vi "Move.vi"(8 "error in (no error)":errorcluster, 11 "IgusMotorDrive in":refnum<class "IgusMotorDrive.lvclass">) -> (0 "error out":errorcluster, 3 "IgusMotorDrive out":refnum<class "IgusMotorDrive.lvclass">)   [LabVIEW 2016, in "IgusMotorDrive.lvclass"]
uses:
  IgusMotorDrive.lvclass
  C:/Users/illogicdev/Desktop/IGUS/IgusPositioningSystem Folder/Modules/Classes/motor-drive/MotorDrive.lvclass
  Libraries/Modbus-Master/MB_PDU/MB_PDU_Cluster.ctl
  typedefs/Controlword--cluster.ctl
  IgusMotorDrive.lvclass/IgusMotorDrive.ctl
  Libraries/Modbus-Master/MB_Master_TCP/MB_Master_TCP.lvclass
  C:/Users/illogicdev/Desktop/IGUS/IgusPositioningSystem Folder/Modules/Libraries/Modbus-Master/MB_Master/MB_Master.lvclass
  motor-drive/MotorDrive.lvclass
  Libraries/Modbus-Master/MB Master.lvlib
panel:
  out "operation mode":u8
  out "Command":T1 {"Data" format="%.0x"}
  out "Response":T1 {"Data" format="%.0x"}
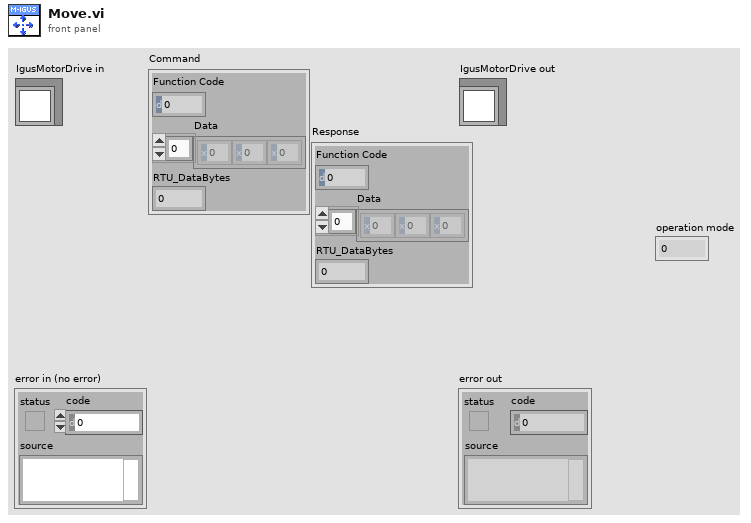
[diagram p1: front panel]
types:
  T1 = typedef "MB Master.lvlib/MB_PDU_Cluster.ctl" = cluster{"Function Code":u8, "Data":u8[], "RTU_DataBytes":i32}
  T2 = typedef "IgusMotorDrive.lvclass/Controlword--cluster.ctl" = cluster{"Switch On":bool, "Enable Voltage":bool, "Quick Stop":bool, "Enable Operation":bool, "4 MS (0: Homing Blocked/1: Homing Start) (0: No Start Signal/1: Start of Movement (0>1))":bool, "5 MS":bool, "6 MS(0:Absolute Positioning/1:Relative Positioning)":bool, "Fault Reset":bool, "Stop":bool, "9 MS":bool, "10 Reserved":bool, "11 Manufacturer Specific":bool, "12 Manufacturer Specific":bool, "13 Manufacturer Specific":bool, "14 Manufacturer Specific":bool, "15 Manufacturer Specific":bool}
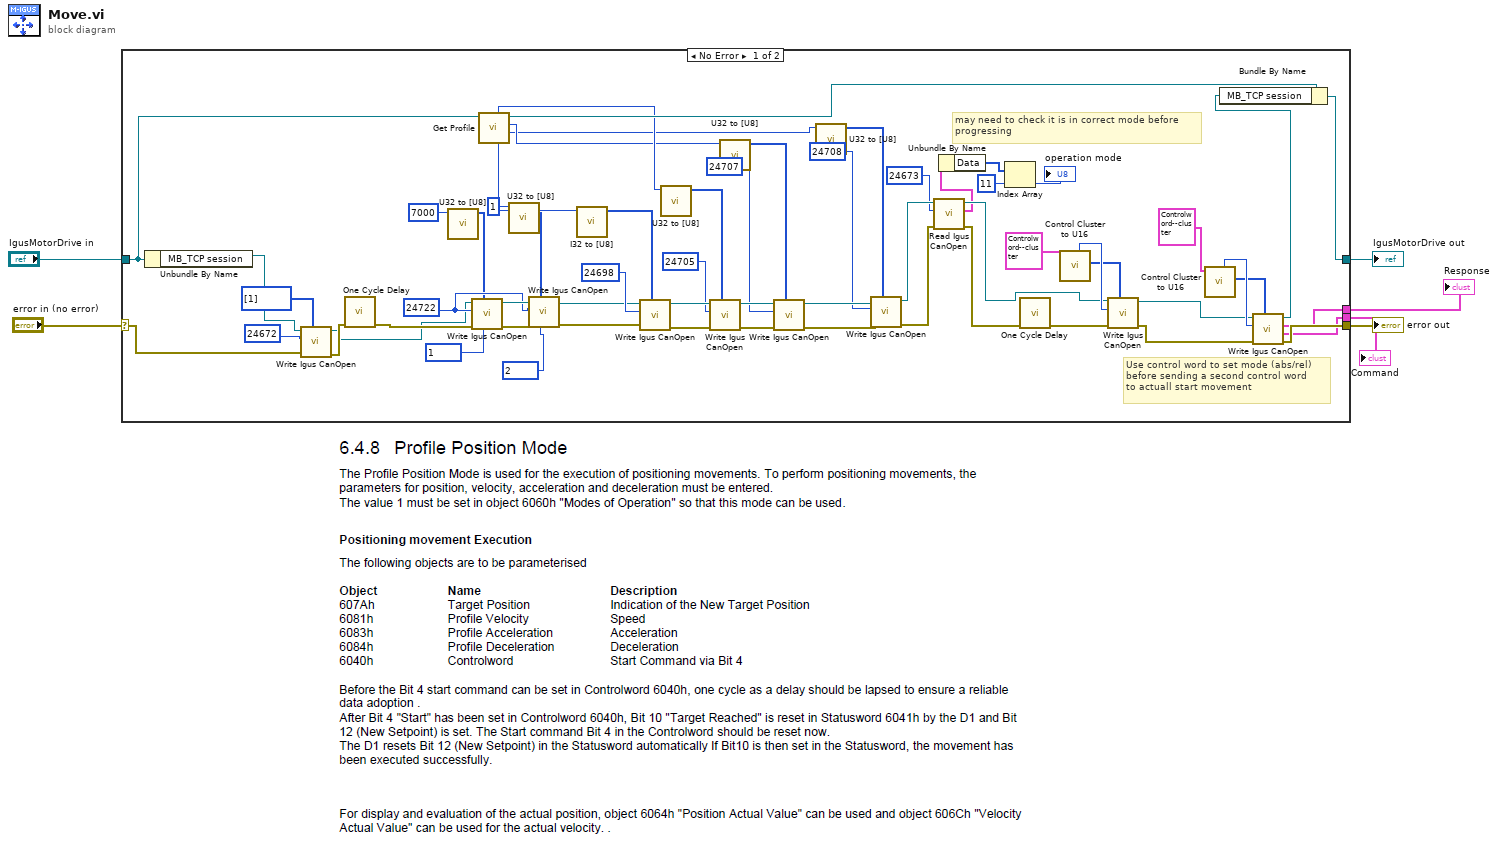
[diagram p0: block diagram]
diagram:
  n1 = case shown="No Error" "error in (no error)" {
    selector: "error in (no error)" -> [w26 w68]
    tunnel: "IgusMotorDrive in" -> [w66 w69]
    tunnel: [w64 w69] -> w4
    tunnel: [w16 w68] -> w3
    tunnel: [w13 _] -> w2
    tunnel: [w12 _] -> w1
    frame No Error {
      w34 = u16 24722 ("address")
      # "Use control word to set mode (abs/rel)\nbefore sending a second control word \nto actuall start movement"
      # "may need to check it is in correct mode before\nprogressing"
      n2 = Unbundle By Name(w66) -> ("MB_TCP session"=w23:refnum<class "MB_Master_TCP.lvclass">)
      n3 = call "Write Igus CanOpen.vi"("Data [1-4]"=u8[] [1], "error in (no error)"=w26, "Address"=u16 24672 ("address"), "MB session in"=w23) -> ("error out"=w25:errorcluster, "MB session out"=w24:refnum<class "MB_Master_TCP.lvclass">)  [unwired: 4 in, 2 out]
      n4 = call "One Cycle Delay.vi"("error in"=w25) -> ("error out"=w31:errorcluster)  [unwired: 10 in]
      n5 = call "U32 to [U8].vi"("Numeric"=u32 7000) -> ("output array"=w32:u8[])  [unwired: 10 in]
      n6 = call "Write Igus CanOpen.vi"("Sub Index"=u8 1 ("address"), "Data [1-4]"=w32, "error in (no error)"=w31, "Address"=w34, "MB session in"=w24) -> ("error out"=w38:errorcluster, "MB session out"=w37:refnum<class "MB_Master_TCP.lvclass">)  [unwired: 3 in, 2 out]
      n7 = call "Get Profile.vi"("MotorDrive in"=w66) -> ("Setpoint Deceleration"=w44:u32, "Setpoint Acceleration"=w49:u32, "MotorDrive out"=w65:refnum<class "IgusMotorDrive.lvclass">, "Setpoint Position"=w62:i32, "Setpoint Velocity"=w53:u32)  [unwired: 5 in, 1 out]
      n8 = call "U32 to [U8].vi"("Numeric"=u32 1) -> ("output array"=w33:u8[])  [unwired: 10 in]
      n9 = call "Write Igus CanOpen.vi"("Sub Index"=u8 2 ("address"), "Data [1-4]"=w33, "error in (no error)"=w38, "Address"=w34, "MB session in"=w37) -> ("error out"=w30:errorcluster, "MB session out"=w29:refnum<class "MB_Master_TCP.lvclass">)  [unwired: 3 in, 2 out]
      n10 = call "I32 to [U8].vi"("Numeric"=w62) -> ("output array"=w61:u8[])  [unwired: 10 in]
      n11 = call "Write Igus CanOpen.vi"("Data [1-4]"=w61, "error in (no error)"=w30, "Address"=u16 24698 ("address"), "MB session in"=w29) -> ("error out"=w54:errorcluster, "MB session out"=w60:refnum<class "MB_Master_TCP.lvclass">)  [unwired: 4 in, 2 out]
      n12 = call "U32 to [U8].vi"("Numeric"=w53) -> ("output array"=w52:u8[])  [unwired: 10 in]
      n13 = call "Write Igus CanOpen.vi"("Data [1-4]"=w52, "error in (no error)"=w54, "Address"=u16 24705 ("address"), "MB session in"=w60) -> ("error out"=w47:errorcluster, "MB session out"=w59:refnum<class "MB_Master_TCP.lvclass">)  [unwired: 4 in, 2 out]
      n14 = call "U32 to [U8].vi"("Numeric"=w49) -> ("output array"=w48:u8[])  [unwired: 10 in]
      n15 = call "Write Igus CanOpen.vi"("Data [1-4]"=w48, "error in (no error)"=w47, "Address"=u16 24707 ("address"), "MB session in"=w59) -> ("error out"=w46:errorcluster, "MB session out"=w58:refnum<class "MB_Master_TCP.lvclass">)  [unwired: 4 in, 2 out]
      n16 = call "U32 to [U8].vi"("Numeric"=w44) -> ("output array"=w43:u8[])  [unwired: 10 in]
      n17 = call "Write Igus CanOpen.vi"("Data [1-4]"=w43, "error in (no error)"=w46, "Address"=u16 24708 ("address"), "MB session in"=w58) -> ("error out"=w39:errorcluster, "MB session out"=w42:refnum<class "MB_Master_TCP.lvclass">)  [unwired: 4 in, 2 out]
      n18 = call "Read Igus CanOpen.vi"("error in (no error)"=w39, "Address"=u16 24673 ("address"), "MB session in"=w42) -> ("error out"=w40:errorcluster, "Response"=w10:T1, "MB session out"=w41:refnum<class "MB_Master_TCP.lvclass">)  [unwired: 5 in, 1 out]
      n19 = Unbundle By Name(w10) -> ("Data"=w9:u8[])
      n20 = Index Array(array=w9, index=11) -> (element=→"operation mode":u8)
      n21 = call "One Cycle Delay.vi"("error in"=w40) -> ("error out"=w55:errorcluster)  [unwired: 10 in]
      n22 = call "Control Cluster to U16.vi"("Controlword"=T2 {"Switch On"=TRUE, "Enable Voltage"=TRUE, "Quick Stop"=TRUE, "Enable Operation"=TRUE, "4 MS (0: Homing Blocked/1: Homing Start) (0: No Start Signal/1: Start of Movement (0>1))"=FALSE, "5 MS"=FALSE, "6 MS(0:Absolute Positioning/1:Relative Positioning)"=FALSE, "Fault Reset"=FALSE, "Stop"=FALSE, "9 MS"=FALSE, "10 Reserved"=FALSE, "11 Manufacturer Specific"=FALSE, "12 Manufacturer Specific"=FALSE, "13 Manufacturer Specific"=FALSE, "14 Manufacturer Specific"=FALSE, "15 Manufacturer Specific"=FALSE}) -> ("Control word Data"=w56:u8[], "address"=w57:u16)  [unwired: 8 in, 1 out]
      n23 = call "Write Igus CanOpen.vi"("Data [1-4]"=w56, "error in (no error)"=w55, "Address"=w57, "MB session in"=w41) -> ("error out"=w18:errorcluster, "MB session out"=w15:refnum<class "MB_Master_TCP.lvclass">)  [unwired: 4 in, 2 out]
      n24 = call "Control Cluster to U16.vi"("Controlword"=T2 {"Switch On"=TRUE, "Enable Voltage"=TRUE, "Quick Stop"=TRUE, "Enable Operation"=TRUE, "4 MS (0: Homing Blocked/1: Homing Start) (0: No Start Signal/1: Start of Movement (0>1))"=TRUE, "5 MS"=FALSE, "6 MS(0:Absolute Positioning/1:Relative Positioning)"=FALSE, "Fault Reset"=FALSE, "Stop"=FALSE, "9 MS"=FALSE, "10 Reserved"=FALSE, "11 Manufacturer Specific"=FALSE, "12 Manufacturer Specific"=FALSE, "13 Manufacturer Specific"=FALSE, "14 Manufacturer Specific"=FALSE, "15 Manufacturer Specific"=FALSE}) -> ("Control word Data"=w19:u8[], "address"=w20:u16)  [unwired: 8 in, 1 out]
      n25 = call "Write Igus CanOpen.vi"("Data [1-4]"=w19, "error in (no error)"=w18, "Address"=w20, "MB session in"=w15) -> ("error out"=w16:errorcluster, "Command"=w12:T1, "Response"=w13:T1, "MB session out"=w14:refnum<class "MB_Master_TCP.lvclass">)  [unwired: 4 in]
      n26 = Bundle By Name(cluster=w65, "MB_TCP session"=w14) -> (w64:refnum<class "IgusMotorDrive.lvclass">)
    }
    frame Error {
    }
  }
  "error out" <- w3
  "IgusMotorDrive out" <- w4
  "Response" <- w2
  "Command" <- w1
